vi "Operator.vi"(8 "error in (no error)":errorcluster, 11 "XBoxController.lvclass":refnum<class "XBoxController.lvclass">) -> (0 "error out":errorcluster)   [LabVIEW 2013]
uses:
  XboxController/XBoxController.lvclass
  XboxController/XBoxController.lvclass/XBoxController.ctl
  <vilib>/Rock Robotics/WPI/Joystick/WPI_JoystickGet.vi
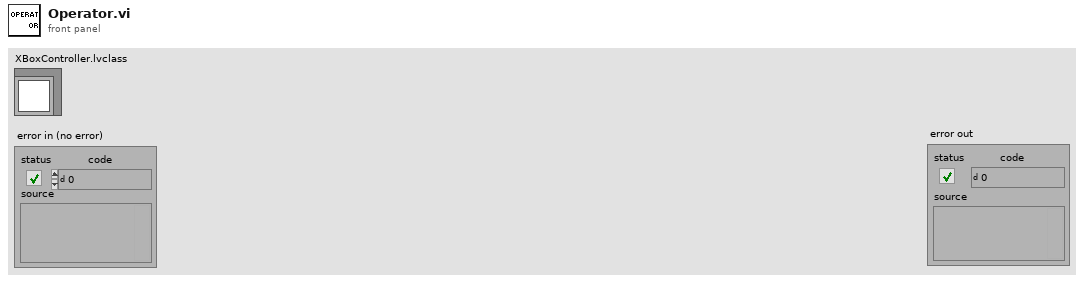
[diagram p1: front panel]
types:
  T1 = typedef "XBoxController.lvclass/Xbox Buttons.ctl" = cluster{"RightBumper":bool, "Left Bumper":bool, "Left Joy Down":bool, "Right Joy Down":bool, "Back":bool, "Start":bool, "D-Pad Left":bool, "D-Pad Right":bool, "Y":bool, "B":bool, "A":bool, "X":bool}
  T2 = cluster{"Left Trigger":dbl, "Right Trigger":dbl, "Left Triggered":bool, "Right Triggered":bool}
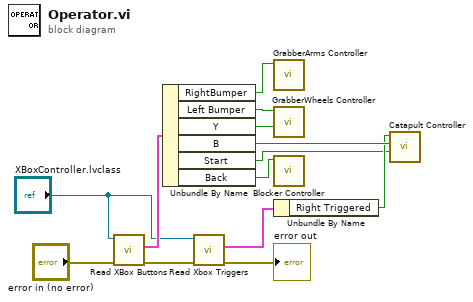
[diagram p0: block diagram]
diagram:
  n1 = call "Read XBox Buttons.vi"("error in (no error)"="error in (no error)", "XBoxController in"="XBoxController.lvclass") -> ("error out"=w7:errorcluster, "XBox Buttons"=w13:T1)  [unwired: 7 in, 1 out]
  n2 = Unbundle By Name(w13) -> ("RightBumper"=w12:bool, "Left Bumper"=w10:bool, "Y"=w9:bool, "B"=w5:bool, "Start"=w2:bool, "Back"=w1:bool)
  n3 = call-dynamic "Read Xbox Triggers.vi"("error in (no error)"=w7, "XBoxController in"="XBoxController.lvclass") -> ("error out"=→"error out":errorcluster, "Xbox Triggers"=w4:T2)  [unwired: 7 in, 1 out]
  n4 = call "GrabberArms Controller.vi"("Extend GrabberArms"=w12) -> ()  [unwired: 10 in, 1 out]
  n5 = call "GrabberWheels Controller.vi"("GW Spit Out"=w9, "GW Full Speed Pickup"=w10) -> ()  [unwired: 9 in, 1 out]
  n6 = call "Blocker Controller.vi"("Blocker Toggle"=w1) -> ()  [unwired: 11 in]
  n7 = Unbundle By Name(w4) -> ("Right Triggered"=w3:bool)
  n8 = call "Catapult Controller.vi"("De-energize w/out Re-energizing"=w2, "Wedge Button"=w5, "Catapult Trigger"=w3) -> ()  [unwired: 8 in, 1 out]
